vi "niFpgaMemorySimulationPathToInit.vi"() -> ()   [LabVIEW 2017]
panel:
  in  "SimulationPathToMemoryInit":string="..\\niFpga\\"
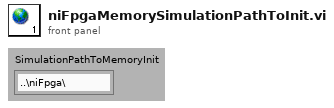
[diagram p1: front panel]
diagram:
